vi "Parse XML Errors.vi"(8 "error in":errorcluster, 11 "XML File Path":path) -> (0 "error out":errorcluster)   [LabVIEW 2021]
doc: "Opens an XML file specified at <b>XML File Path</b> input and tries to parse it. The XML file has to be in format of XML file which is generated by LabVIEW build-in Error Code Editor (Tools->Advanced->Edit Error Codes...)\nThe error code and error description is extracted at this XPATHs:\n<b>Error Code:</b> /nidocument/nierror/@code\n<b>Error Description:</b> /nidocument/nierror\n\nParsed error code and description is inserted into map structure, where key is the error ID and value is the error description. Map containing errors elements is stored in FGV Map of Errors variable."
uses:
  <vilib>/xml/Close Reference(Node).vi
  <vilib>/xml/NI_XML.lvlib
  <resource>/objmgr/DOMUserDefRef.rc
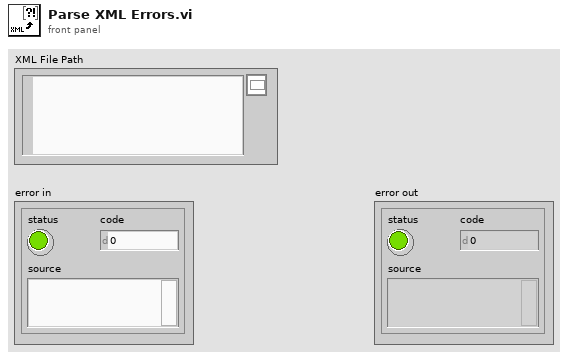
[diagram p1: front panel]
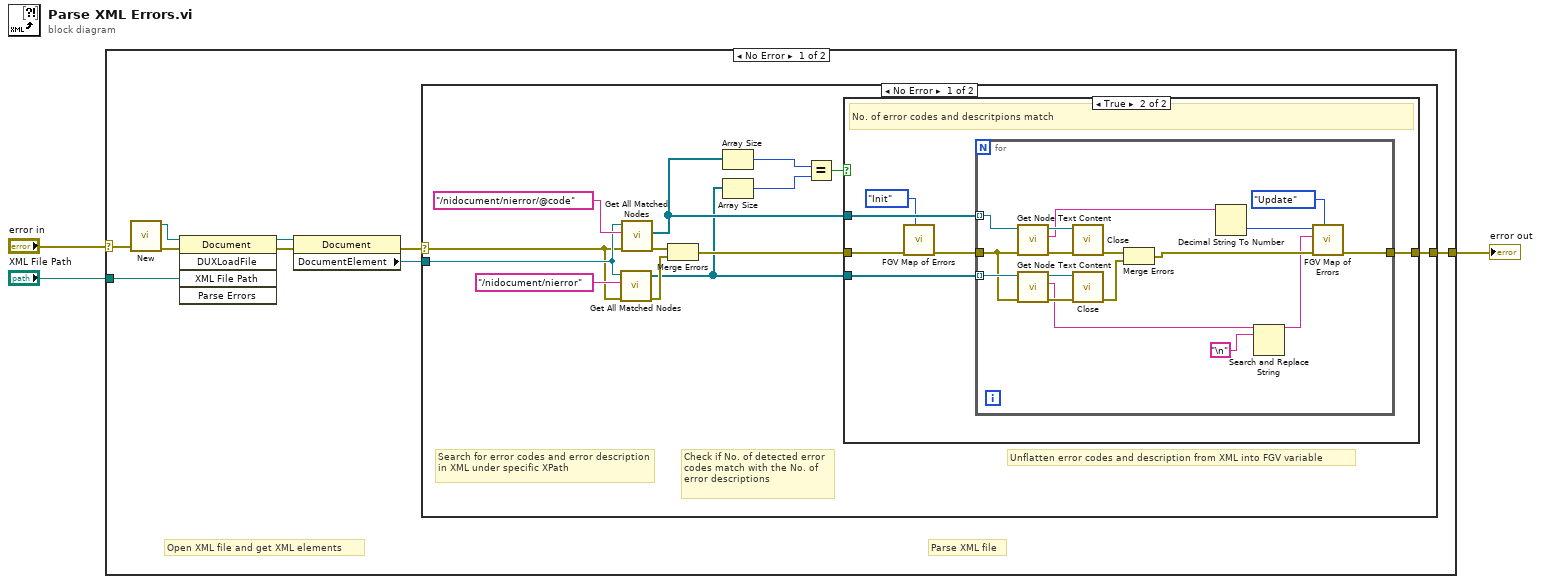
[diagram p0: block diagram]
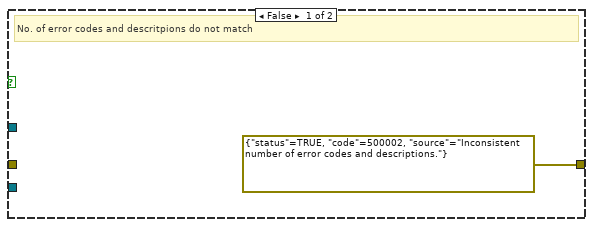
[diagram p2: hidden frame]
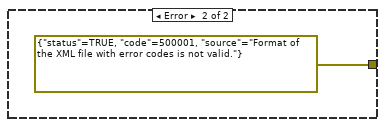
[diagram p3: hidden frame]
diagram:
  n1 = case shown="No Error" "error in" {
    selector: "error in" -> [w5 w51]
    tunnel: "XML File Path" -> [w10 _]
    tunnel: [w6 w51] -> w2
    frame No Error {
      # "Parse XML file"
      # "Open XML file and get XML elements"
      n2 = call <vilib>:"New.vi"("error in (no error)"=w5) -> ("error out"=w11:errorcluster, "DOM document out"=w12:refnum<k20>)  [unwired: 7 in]
      n3 = invoke class="Document" method="DUXLoadFile"(reference=w12, error in=w11, "XML File Path"=w10) -> (reference out=w8:refnum<k20>, error out=w7:errorcluster)  [unwired: 2 in, 3 out]
      n4 = property class="Document"(reference=w8, error in=w7) -> (error out=w4:errorcluster, "DocumentElement"=w9:refnum<k20>)  [unwired: 1 out]
      n5 = case shown="No Error" w4 {
        selector: w4 -> [w13 _]
        tunnel: w9 -> [w23 _]
        tunnel: [w20 errorcluster {"status"=TRUE, "code"=500001, "source"="Format of the XML file with error codes is not valid."} ("error out")] -> w6
        frame No Error {
          # "Unflatten error codes and description from XML into FGV variable"
          # "Check if No. of detected error codes match with the No. of error descriptions"
          # "Search for error codes and error description in XML under specific XPath"
          n6 = call <vilib>:"Get All Matched Nodes.vi"("error in (no error)"=w13, "XPath expression"="/nidocument/nierror", "node in"=w23) -> ("error out"=w22:errorcluster, "node result array"=w17:refnum<k20>[])  [unwired: 6 in, 1 out]
          n7 = call <vilib>:"Get All Matched Nodes.vi"("error in (no error)"=w13, "XPath expression"="/nidocument/nierror/@code", "node in"=w23) -> ("error out"=w24:errorcluster, "node result array"=w18:refnum<k20>[])  [unwired: 6 in, 1 out]
          n8 = Merge Errors(w24, w22) -> (w19:errorcluster)
          n9 = Array Size(array=w18) -> (size(s)=w15:i32)
          n10 = Array Size(array=w17) -> (size(s)=w14:i32)
          n11 = Equal?(x=w15, y=w14) -> (x = y?=w16:bool)
          n12 = case shown="True" w16 {
            tunnel: w18 -> [_ w32]
            tunnel: w17 -> [_ w31]
            tunnel: [errorcluster {"status"=TRUE, "code"=500002, "source"="Inconsistent number of error codes and descriptions."} ("error IO") w30] -> w20
            tunnel: w19 -> [_ w29]
            frame False {
              # "No. of error codes and descritpions do not match"
            }
            frame True {
              # "No. of error codes and descritpions match"
              n13 = call "FGV Map of Errors.vi"("Operation (Get)"=enum16{"Init", "Get", "Update"}."Init", "error in"=w29) -> ("error out"=w28:errorcluster)  [unwired: 8 in, 1 out]
              n14 = for {
                tunnel: w32 -> [w44] mode=indexing
                tunnel: w31 -> [w43] mode=indexing
                tunnel: w28 -> [w42]
                tunnel: [w38] -> w30
                n15 = call <vilib>:"Get Node Text Content.vi"("error in (no error)"=w42, "node in"=w44) -> ("error out"=w48:errorcluster, "node text"=w40:string, "node out"=w47:refnum<k20>)  [unwired: 7 in]
                n16 = call <vilib>:"Get Node Text Content.vi"("error in (no error)"=w42, "node in"=w43) -> ("error out"=w45:errorcluster, "node text"=w39:string, "node out"=w46:refnum<k20>)  [unwired: 7 in]
                n17 = call-poly <vilib>:"Close.vi"("error in (no error)"=w48, "node"=w47) -> ("error out"=w49:errorcluster)  [unwired: 7 in]
                n18 = call-poly <vilib>:"Close.vi"("error in (no error)"=w45, "node"=w46) -> ("error out"=w41:errorcluster)  [unwired: 7 in]
                n19 = Merge Errors(w49, w41) -> (w37:errorcluster)
                n20 = Decimal String To Number(string=w40) -> (number=w34:i32)  [unwired: 2 in, 1 out]
                n21 = Search and Replace String(input string=w39, search string="\n") -> (result string=w33:string)  [unwired: 6 in, 3 out]
                n22 = call "FGV Map of Errors.vi"("Operation (Get)"=enum16{"Init", "Get", "Update"}."Update", "error in"=w37, "error description"=w33, "error code"=w34) -> ("error out"=w38:errorcluster)  [unwired: 6 in, 1 out]
              }
            }
          }
        }
        frame Error {
        }
      }
    }
    frame Error {
    }
  }
  "error out" <- w2
